vi "SCMP pic gen.vi"(10 "Height":i64, 11 "Width":i64) -> (2 "demo image":u16[](array[numeric]), 3 "Intensity Graph":u8[][](graph))   [LabVIEW 2014]
panel:
  out "path":path
  out "2D Picture":picture
  out "Intensity Graph 2":u16[][](graph)
  out "width":i16
  out "hight":i16
  out "Image Data":u16[][](array[numeric])
  out "Image":u16[][](graph)
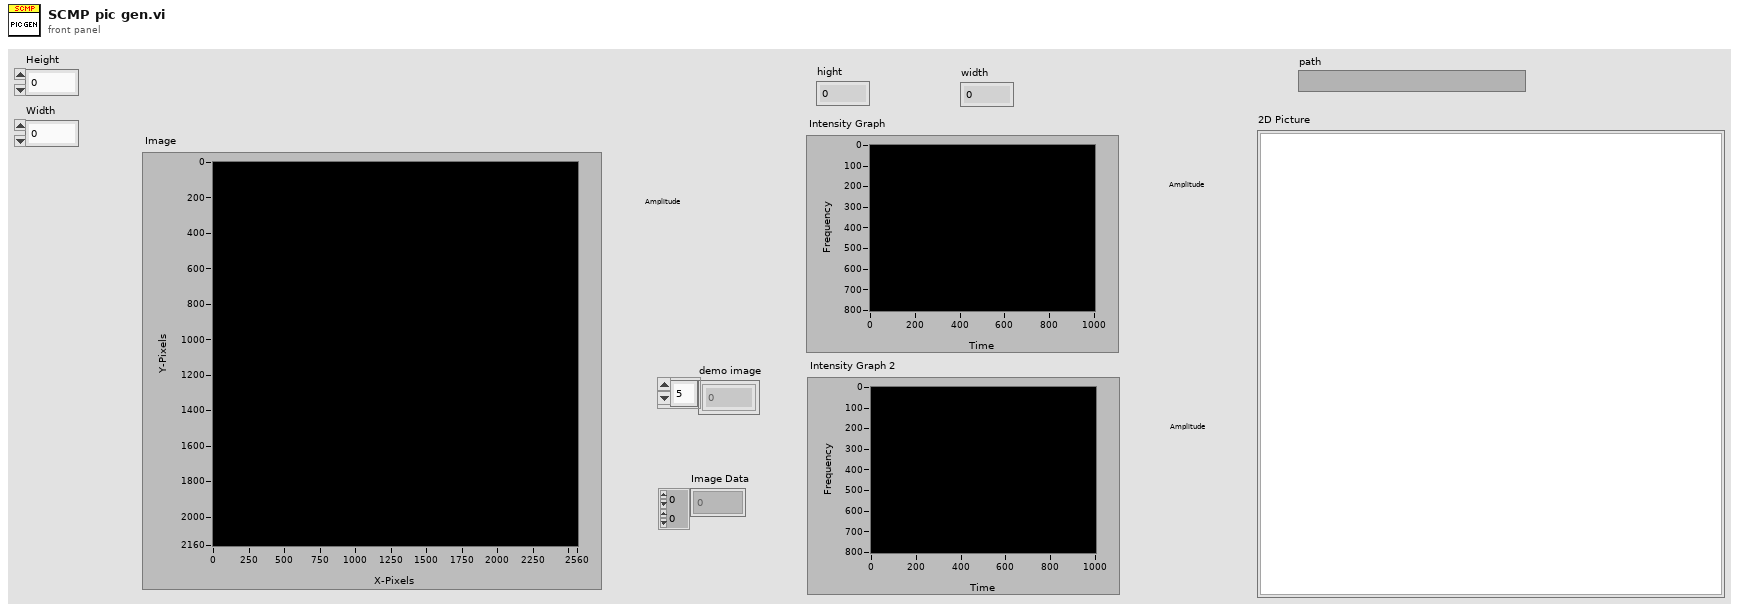
[diagram p1: front panel]
types:
  T1 = cluster{"Font Name:":string, "Size":i16, "Strikeout?":bool, "Italic?":bool, "Underline?":bool, "Outline?":bool, "Shadow?":bool, "Bold?":bool}
  T2 = enum16{"User-specified Font", "Application Font", "System Font", "Dialog Font"}
  T3 = cluster{"left":i16, "top":i16, "right":i16, "bottom":i16}
  T4 = typedef "imagedata.ctl" = cluster{"image type":i32, "image depth":i32, "image":u8[], "mask":u8[], "colors":u32[], "Rectangle":cluster{"left":i16, "top":i16, "right":i16, "bottom":i16}}
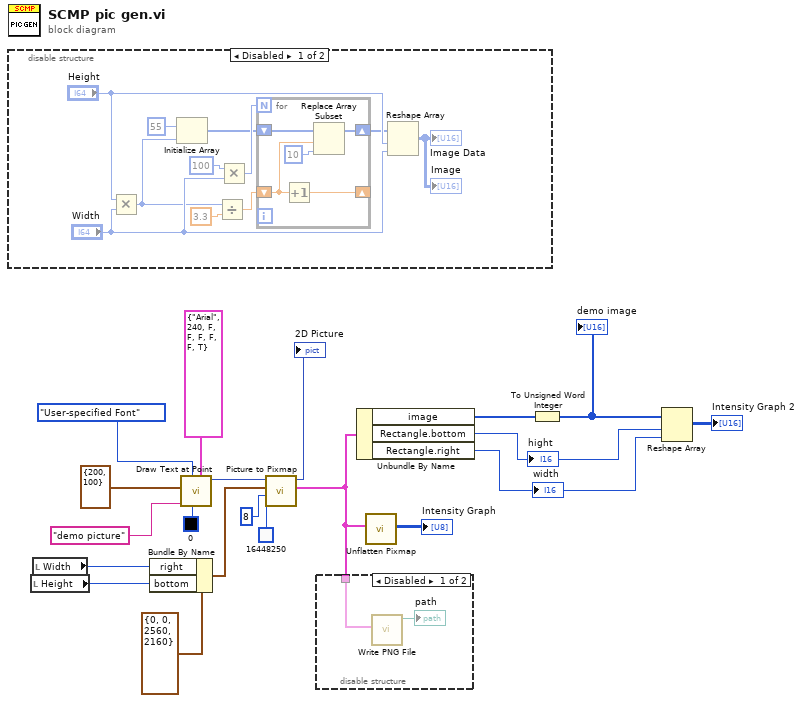
[diagram p0: block diagram]
diagram:
  n1 = disable-structure shown="Disabled" {
    frame Disabled {
      n2 = Multiply(x="Height", y="Width") -> (x*y=w24:i64)
      n3 = Initialize Array(u16 55 ("element"), w24) -> (w26:u16[])
      n4 = Divide(x=w24, y=3.3) -> (x/y=w23:dbl)
      n5 = Multiply(x=i64 100, y="Width") -> (x*y=w29:i64)
      n6 = for {
        N: w29 -> [_]
        shift-right: [w35] -> w21
        shift-left: w26 -> [w36]
        shift-right: [w32] -> _
        shift-left: w23 -> [w33]
        n7 = Increment(x=w33) -> (x+1=w32:dbl)
        n8 = Replace Array Subset(array=w36, new element=u16 10 ("new element/subarray"), index=w33) -> (w35:u16[])
      }
      n9 = Reshape Array(w21, "Height", "Width") -> (→"Image" →"Image Data":u16[][])
    }
    frame Enabled {
    }
  }
  n10 = local read "Height"() -> (w6:i64)
  n11 = local read "Width"() -> (w5:i64)
  n12 = Bundle By Name(cluster=T3 {"left"=0, "top"=0, "right"=2560, "bottom"=2160} ("rect"), "right"=w5, "bottom"=w6) -> (w7:T3)
  n13 = call <vilib>:"Draw Text at Point.vi"("[user-specified font]"=T1 {"Font Name:"="Arial", "Size"=240, "Strikeout?"=FALSE, "Italic?"=FALSE, "Underline?"=FALSE, "Outline?"=FALSE, "Shadow?"=FALSE, "Bold?"=TRUE}, "text color(black)"=u32 0, "desired font(Application)"=T2."User-specified Font", "text"="demo picture", "origin"=cluster{"x":i16, "y":i16} {"x"=200, "y"=100}) -> ("new picture"=w18:picture)  [unwired: 5 in, 1 out]
  n14 = call <vilib>:"Picture to Pixmap.vi"("Background Color"=u32 16448250, "depth"=8, "rect"=w7, "picture"=w18) -> ("image data"=w1:T4, "new picture"=→"2D Picture":picture)  [unwired: 6 in]
  n15 = disable-structure shown="Disabled" {
    disable-tunnel: w1 -> [w38 _]
    frame Disabled {
      n16 = call <vilib>:"Write PNG File.vi"("image data"=w38) -> ("path"=→"path":path)  [unwired: 9 in, 1 out]
    }
    frame Enabled {
    }
  }
  n17 = Unbundle By Name(w1) -> ("image"=w9:u8[], "Rectangle.bottom"=w12:i16, "Rectangle.right"=w2:i16)
  "hight" <- w12
  "width" <- w2
  n18 = call <vilib>:"Unflatten Pixmap.vi"("image data"=w1) -> ("8-bit pixmap"=→"Intensity Graph":u8[][])  [unwired: 4 in, 6 out]
  n19 = To Unsigned Word Integer(number=w9) -> (unsigned 16bit integer=w8:u16[])
  "demo image" <- w8
  n20 = Reshape Array(w8, w12, w2) -> (→"Intensity Graph 2":u16[][])
